vi "EjemploMaquinaEstadosFinitos.vi"() -> ()   [LabVIEW 2020]
panel:
  out "Alarma":bool
  in  "Limite":dbl
  out "Historiador":dynamicdata(graph)
  in  "Temperatura gC":dbl(slide) scale=0.0..100.0
  in  "stop":bool
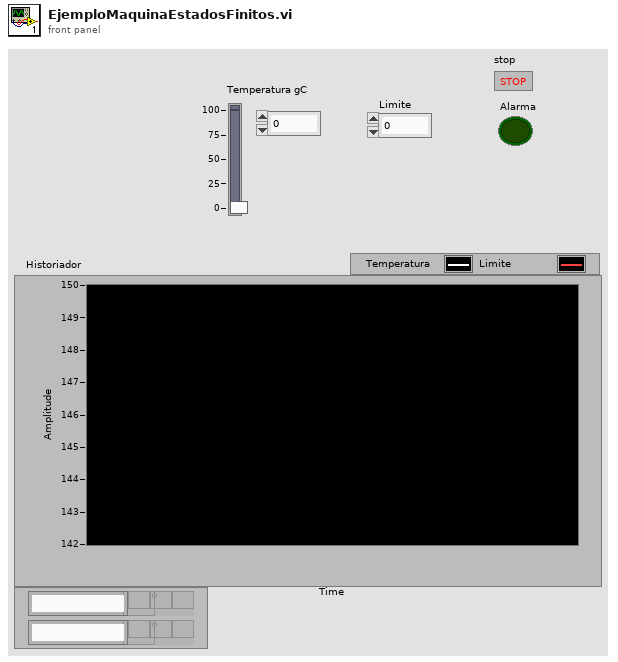
[diagram p1: front panel]
types:
  T1 = enum16{"Estado_Inicio", "Alarma_On", "Alarma_Off", "Retardo", "DAQ"}
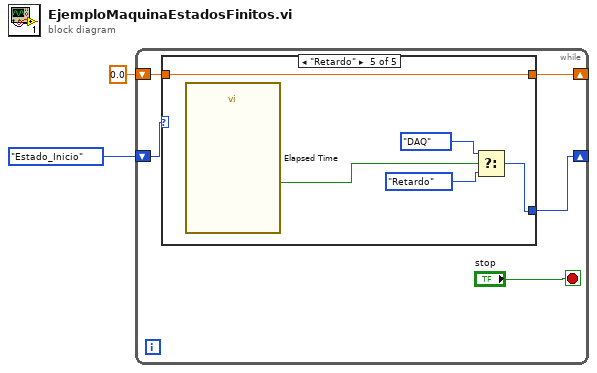
[diagram p0: block diagram]
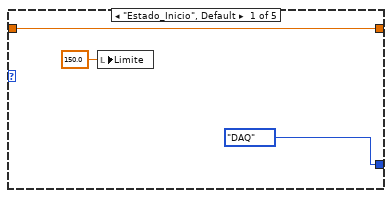
[diagram p2: hidden frame]
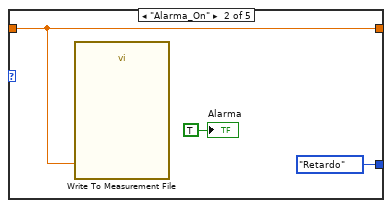
[diagram p3: hidden frame]
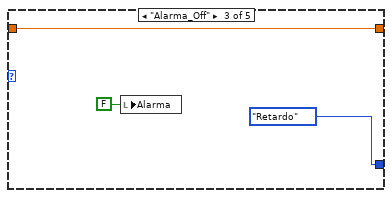
[diagram p4: hidden frame]
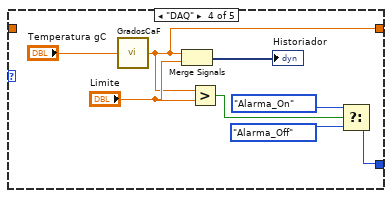
[diagram p5: hidden frame]
diagram:
  n1 = while {
    shift-right: [w6] -> _
    shift-left: 0.0 ("Temperatura gF") -> [w5]
    shift-right: [w3] -> _
    shift-left: T1."Estado_Inicio" ("Estados") -> [w4]
    stop <- "stop" stop-if-true
    n2 = case shown="\"Retardo\"" w4 {
      tunnel: [w10 w12 w16 w18 w29] -> w6
      tunnel: w5 -> [w10 w12 w16 _ w29]
      tunnel: [T1."DAQ" ("Estados") T1."Retardo" ("Estados") T1."Retardo" ("Estados") w17 w25] -> w3
      frame "Estado_Inicio", Default {
        n3 = local write "Limite"(150.0 ("Limite")) -> ()
      }
      frame "Alarma_On" {
        n4 = call "Write To Measurement File"("Signals"=w12) -> ()  [unwired: 16 in, 3 out]
        "Alarma" <- TRUE ("Alarma")
      }
      frame "Alarma_Off" {
        n5 = local write "Alarma"(FALSE ("Alarma")) -> ()
      }
      frame "DAQ" {
        n6 = call "GradosCaF.vi"("Temperatura gC"="Temperatura gC") -> ("Temperatura gF"=w18:dbl)
        n7 = Merge Signals(w18, "Limite") -> (→"Historiador":dynamicdata)
        n8 = Greater?(x=w18, y="Limite") -> (0:w21:bool)
        n9 = Select(t=T1."Alarma_On" ("Estados"), s=w21, f=T1."Alarma_Off" ("Estados")) -> (s? t:f=w17:T1)
      }
      frame "Retardo" {
        n10 = call "Elapsed Time"() -> ("Time has Elapsed"=w28:bool)  [unwired: 12 in, 7 out]
        n11 = Select(t=T1."DAQ" ("Estados"), s=w28, f=T1."Retardo" ("Estados")) -> (s? t:f=w25:T1)
      }
    }
  }
